vi "Definition Cluster.vi"(11 "Text in":refnum<class "Text.lvclass">) -> (2 "Definition":variant, 3 "Text out":refnum<class "Text.lvclass">)   [LabVIEW 2020, in "Conditum.lvlib" / "Columns.lvlib" / "Text.lvclass"]
uses:
  Text.lvclass
  Text.lvclass/Text.ctl
  Attributes.ctl
  Conditum.lvlib
  Type/Definition.ctl
  Type/Type.lvclass
  Definition.ctl
  Text Definition.ctl
  C:/dev/lv20CE/lv-conditum/Conditum/Columns/Type/Type.lvclass
  C:/dev/lv20CE/lv-conditum/Conditum/Columns/Text/Text.lvclass
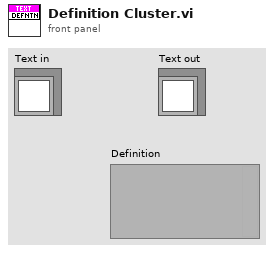
[diagram p1: front panel]
types:
  T1 = typedef "Conditum.lvlib/Columns.lvlib/Text.lvclass/Text Definition.ctl" = cluster{"Type":T2, "Attributes":T3, "Text":T4}
  T2 = typedef "Conditum.lvlib/Columns.lvlib/Type.lvclass/Definition.ctl" = cluster{"Name":string, "Nullable":bool, "Default NULL":bool}
  T3 = typedef "Conditum.lvlib/Attributes.ctl" = cluster{"Primary Key":bool, "Unique":bool, "Foreign Key":bool, "Auto Increment":bool}
  T4 = typedef "Conditum.lvlib/Columns.lvlib/Text.lvclass/Definition.ctl" = cluster{"Default":string}
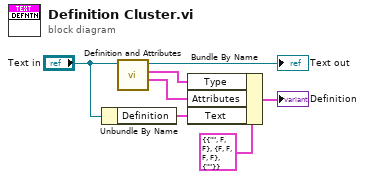
[diagram p0: block diagram]
diagram:
  n1 = Unbundle By Name("Text in") -> ("Definition"=w6:T4)
  n2 = call "Definition and Attributes.vi"("Type in"="Text in") -> ("Attributes"=w4:T3, "Definition"=w5:T2, "Type out"=→"Text out":refnum<class "Text.lvclass">)  [unwired: 8 in]
  n3 = Bundle By Name(cluster=T1 {"Type"={"Name"="", "Nullable"=FALSE, "Default NULL"=FALSE}, "Attributes"={"Primary Key"=FALSE, "Unique"=FALSE, "Foreign Key"=FALSE, "Auto Increment"=FALSE}, "Text"={"Default"=""}} ("Definition"), "Type"=w5, "Attributes"=w4, "Text"=w6) -> (→"Definition":T1)
